vi "Test2.vi"() -> ()   [LabVIEW 2014]
panel:
  out "FrameIn":u8[](array[numeric])
  out "FrameNak":u8[](array[numeric])
  out "XY Graph":cluster{i32[], i32[]}(graph)
  in  "error out":errorcluster
  out "String":string="Coś się zjebało"
  out "Enum":T1(ring)
  in  "stop while":bool
  in  "Stop":bool
  out "SerialNumber":string
  out "Information":string
  in  "Start":bool
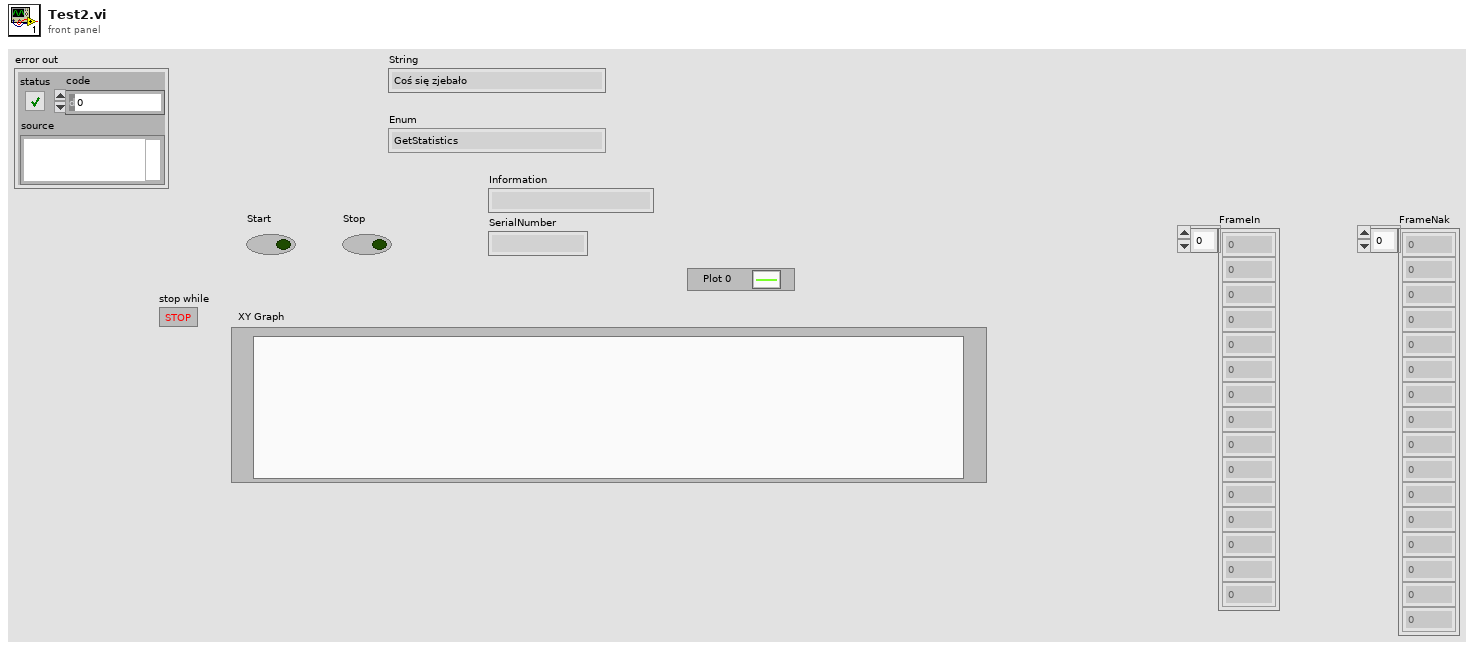
[diagram p1: front panel]
types:
  T1 = enum16{"GetStatistics", "StartAcquisition", "FindAnalyzer", "Start", "Stop"}
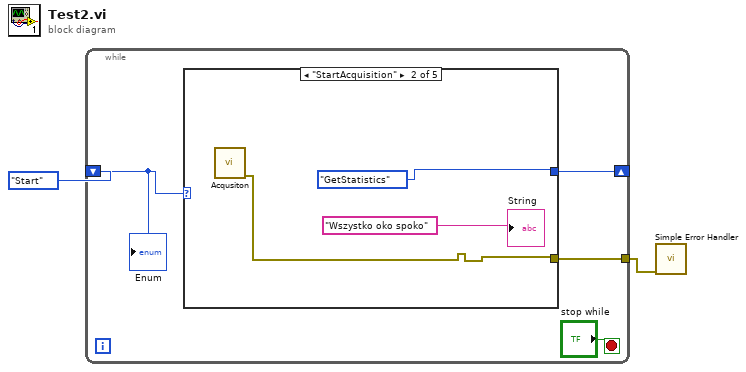
[diagram p0: block diagram]
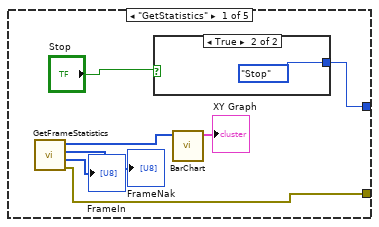
[diagram p2: hidden frame]
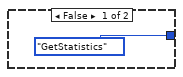
[diagram p3: hidden frame]
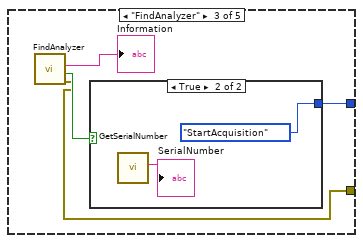
[diagram p4: hidden frame]
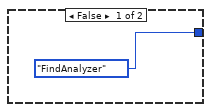
[diagram p5: hidden frame]
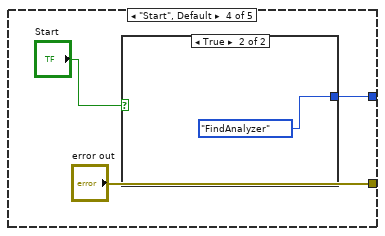
[diagram p6: hidden frame]
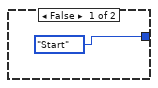
[diagram p7: hidden frame]
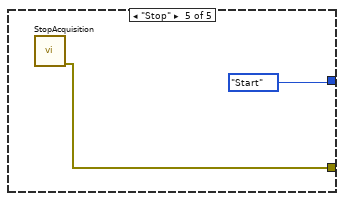
[diagram p8: hidden frame]
diagram:
  n1 = while {
    shift-right: [w5] -> _
    shift-left: T1."Start" ("Enum") -> [w6]
    tunnel: [w3] -> w1
    stop <- "stop while" stop-if-true
    n2 = case shown="\"StartAcquisition\"" w6 {
      tunnel: [w12 T1."GetStatistics" ("Enum") w20 w27 T1."Start" ("Enum")] -> w5
      tunnel: [w7 w16 w19 "error out" w31] -> w3
      frame "GetStatistics" {
        n3 = call "GetFrameStatistics.vi"() -> ("error out"=w7:errorcluster, "FrameIn"=→"FrameIn":u8[], "FrameNak"=→"FrameNak":u8[], "FrameOut"=w11:u8[])  [unwired: 8 in]
        n4 = case shown="True" "Stop" {
          tunnel: [T1."GetStatistics" ("Enum") T1."Stop" ("Enum")] -> w12
          frame False {
          }
          frame True {
          }
        }
        n5 = call "BarChart.vi"("Array"=w11) -> ("XY Graph"=→"XY Graph":cluster{i32[], i32[]})  [unwired: 9 in, 1 out]
      }
      frame "StartAcquisition" {
        n6 = call "Acqusiton.vi"() -> ("error out"=w16:errorcluster)  [unwired: 10 in, 1 out]
        "String" <- "Wszystko oko spoko"
      }
      frame "FindAnalyzer" {
        n7 = call "FindAnalyzer.vi"() -> ("error out"=w19:errorcluster, "IsFound"=w21:bool, "Information"=→"Information":string)  [unwired: 9 in]
        n8 = case shown="True" w21 {
          tunnel: [T1."FindAnalyzer" ("Enum") T1."StartAcquisition" ("Enum")] -> w20
          frame False {
          }
          frame True {
            n9 = call "GetSerialNumber.vi"() -> ("SerialNumber"=→"SerialNumber":string)  [unwired: 10 in, 1 out]
          }
        }
      }
      frame "Start", Default {
        n10 = case shown="True" "Start" {
          tunnel: [T1."Start" ("Enum") T1."FindAnalyzer" ("Enum")] -> w27
          frame False {
          }
          frame True {
          }
        }
      }
      frame "Stop" {
        n11 = call "StopAcquisition.vi"() -> ("error out"=w31:errorcluster)  [unwired: 10 in, 1 out]
      }
    }
    "Enum" <- w6
  }
  n12 = call <vilib>:"Simple Error Handler.vi"("error in (no error)"=w1) -> ()  [unwired: 4 in, 5 out]
